vi "LINC Create Command Definition.vi"(8 "error in (no error)":errorcluster, 10 "path":path, 11 "LINC session":refnum<class "LINC.lvclass">) -> (0 "error out":errorcluster, 3 "dup LINC session":refnum<class "LINC.lvclass">)   [LabVIEW 2018, in "STEPkgDriver_LINC.lvlib" / "LINC.lvclass"]
uses:
  LINC.lvclass
  STEPkgDriver_LINC.lvlib
  LINC Global Mode.ctl
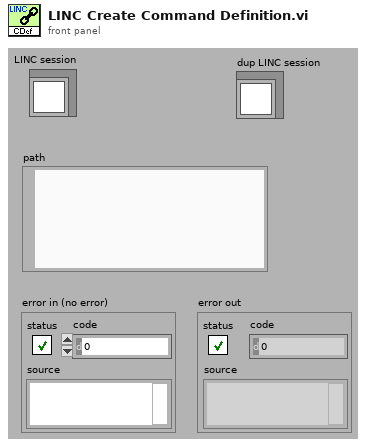
[diagram p1: front panel]
types:
  T1 = typedef "STEPkgDriver_LINC.lvlib/LINC Global Mode.ctl" = enum16{"INIT", "CLEAR", "ADD_PKT_HDR", "ADD_PKT", "GET_PKT_NAMES", "GET_PKT_DESC", "GET_PKT_HDR", "GET_PKT", "SET_PKT", "SET_DATA", "SIM_EN", "SIM_DS"}
  T2 = typedef "STEPkgDriver_LINC.lvlib/LINC Format Prototype.ctl" = cluster{"type":string, "bit offset":i32, "bit size":i32, "format":string, "unit":string, "description":string, "state values":i64[], "states":string[], "max":string, "min":string, "default":string, "array":bool, "bit element size":i32, "poly bound":dbl[], "poly scale":cluster{"coefficients":dbl[]}[], "labview size":i32, "simulate":bool, "ID":bool, "required":bool}
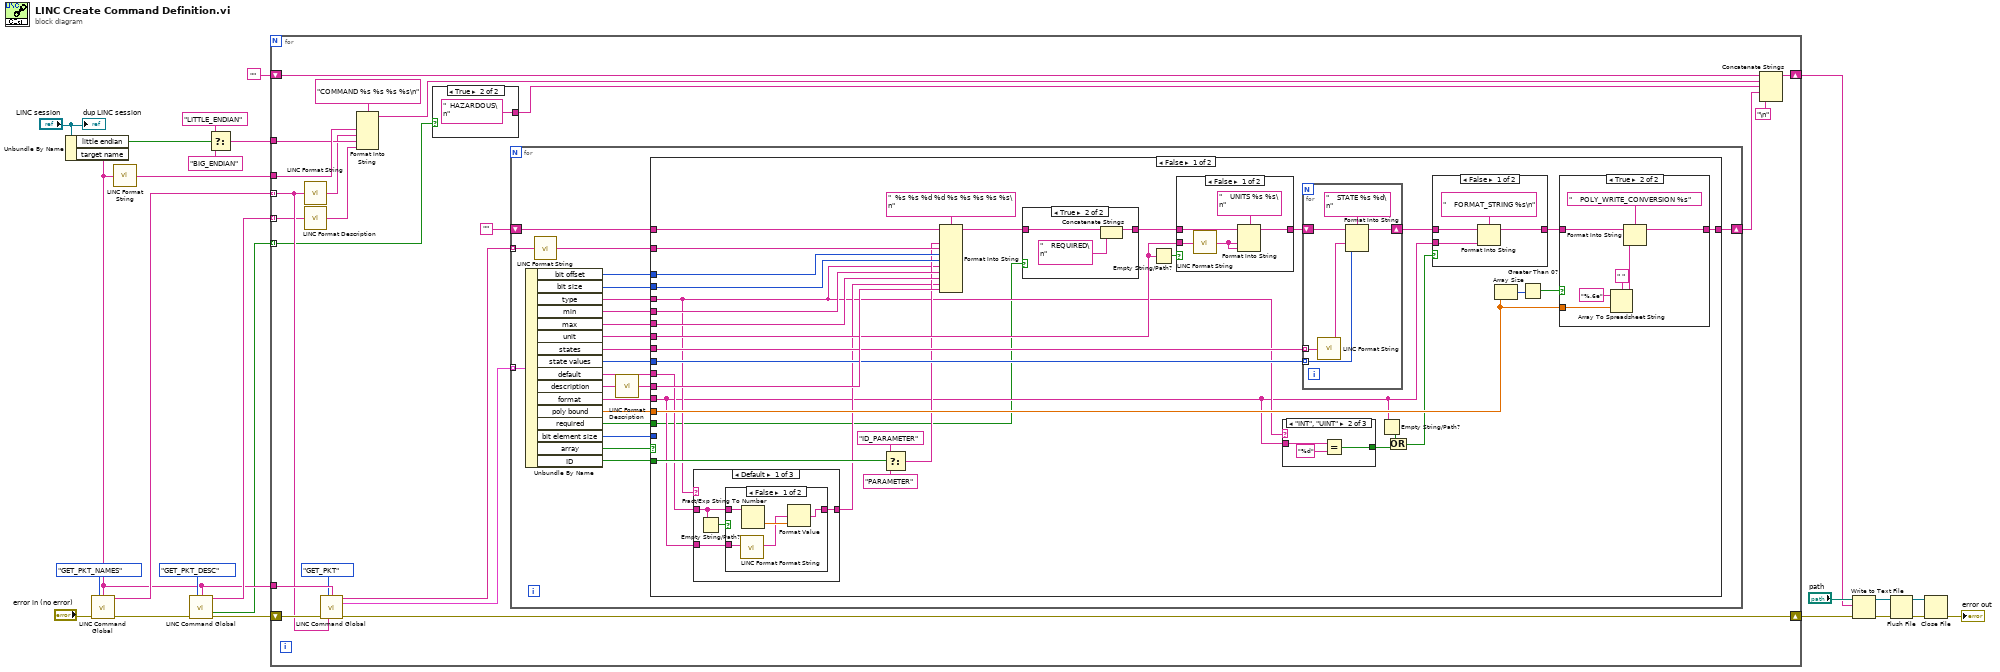
[diagram p0: block diagram]
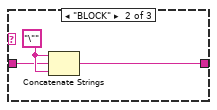
[diagram p5: hidden frame]
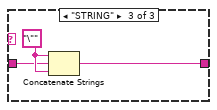
[diagram p6: hidden frame]
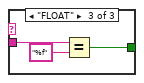
[diagram p8: hidden frame]
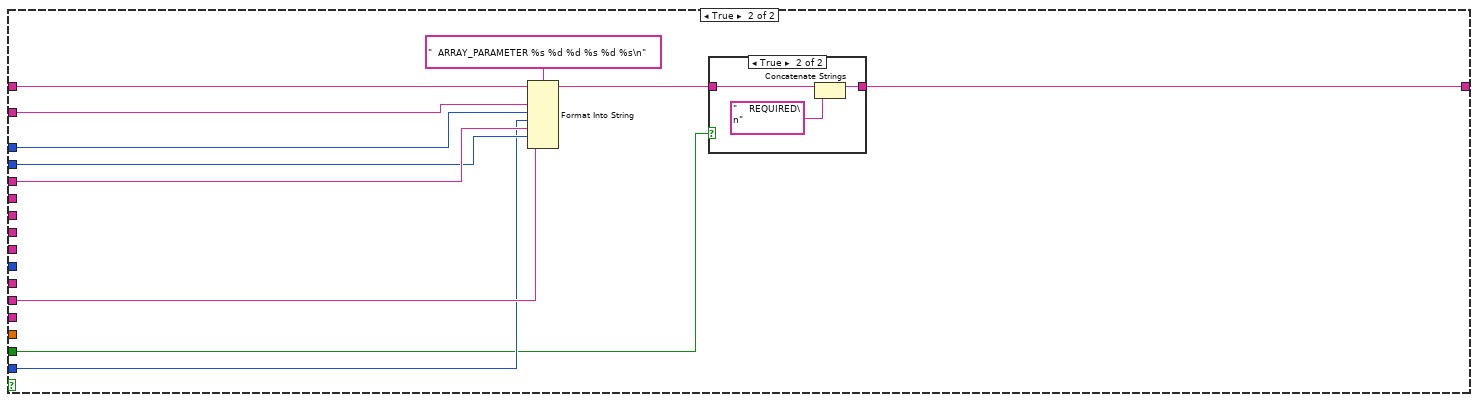
[diagram p12: hidden frame]
diagram:
  n1 = Unbundle By Name("LINC session") -> ("little endian"=w4:bool, "target name"=w2:string)
  n2 = call "LINC Command Global.vi"("mode"=LINC_Global_Mode."GET_PKT_NAMES", "target name"=w2, "error in (no error)"="error in (no error)") -> ("values out"=w17:string[], "error out"=w14:errorcluster)  [unwired: 8 in, 3 out]
  n3 = call "LINC Format String.vi"("string in"=w2) -> ("string out"=w3:string)
  n4 = call "LINC Command Global.vi"("mode"=LINC_Global_Mode."GET_PKT_DESC", "target name"=w2, "error in (no error)"=w14) -> ("values out"=w13:string[], "hazardous out"=w1:bool[], "error out"=w9:errorcluster)  [unwired: 8 in, 2 out]
  n5 = Select(t="LITTLE_ENDIAN", s=w4, f="BIG_ENDIAN") -> (s? t:f=w5:string)
  n6 = for {
    tunnel: w3 -> [w45]
    tunnel: w13 -> [w26] mode=indexing
    shift-right: [w36] -> w8
    shift-left: "" -> [w41]
    shift-right: [w39] -> w16
    shift-left: w9 -> [w40]
    tunnel: w17 -> [w30] mode=indexing
    tunnel: w2 -> [w38]
    tunnel: w5 -> [w32]
    tunnel: w1 -> [w29] mode=indexing
    n7 = call "LINC Format String.vi"("string in"=w30) -> ("string out"=w31:string)
    n8 = call "LINC Format Description.vi"("string in"=w26) -> ("string out"=w25:string)
    n9 = call "LINC Command Global.vi"("mode"=LINC_Global_Mode."GET_PKT", "target name"=w38, "error in (no error)"=w40, "packet name"=w30) -> ("values out"=w34:string[], "item formats out"=w35:T2[], "error out"=w39:errorcluster)  [unwired: 7 in, 2 out]
    n10 = Format Into String(format string="COMMAND %s %s %s %s\n", w45, w31, w32, w25) -> (resulting string=w28:string)  [unwired: 2 in, 1 out]
    n11 = case shown="True" w29 {
      tunnel: [_ "  HAZARDOUS\n" ("format string")] -> w27
      frame False {
      }
      frame True {
      }
    }
    n12 = for {
      shift-right: [w67] -> w37
      shift-left: "" -> [w68]
      tunnel: w34 -> [w50] mode=indexing
      tunnel: w35 -> [w63] mode=indexing
      n13 = Unbundle By Name(w63) -> ("bit offset"=w60:i32, "bit size"=w59:i32, "type"=w64:string, "min"=w56:string, "max"=w55:string, "unit"=w66:string, "states"=w65:string[], "state values"=w62:i64[], "default"=w48:string, "description"=w52:string, "format"=w53:string, "poly bound"=w57:dbl[], "required"=w47:bool, "bit element size"=w58:i32, "array"=w61:bool, "ID"=w54:bool)
      n14 = call "LINC Format String.vi"("string in"=w50) -> ("string out"=w49:string)
      n15 = call "LINC Format Description.vi"("string in"=w52) -> ("string out"=w51:string)
      n16 = case shown="False" w61 {
        tunnel: w68 -> [w100 w162]
        tunnel: [w72 w154] -> w67
        tunnel: w53 -> [w73 _]
        tunnel: w51 -> [w98 w161]
        tunnel: w56 -> [w95 _]
        tunnel: w55 -> [w94 _]
        tunnel: w66 -> [w93 _]
        tunnel: w65 -> [w92 _]
        tunnel: w49 -> [w84 w160]
        tunnel: w64 -> [w75 w159]
        tunnel: w60 -> [w91 w158]
        tunnel: w62 -> [w90 _]
        tunnel: w59 -> [w89 w157]
        tunnel: w58 -> [_ w156]
        tunnel: w57 -> [w85 _]
        tunnel: w54 -> [w83 _]
        tunnel: w48 -> [w74 _]
        tunnel: w47 -> [w69 w153]
        frame False {
          n17 = case shown="Default" w75 {
            tunnel: w74 -> [w108 w117 w120]
            tunnel: [w107 w116 w119] -> w78
            tunnel: w73 -> [w106 _ _]
            frame Default {
              n18 = Empty String/Path?(string/path=w108) -> (empty?=w109:bool)
              n19 = case shown="False" w109 {
                tunnel: w106 -> [w114 _]
                tunnel: w108 -> [w113 w115]
                tunnel: [w110 w115] -> w107
                frame False {
                  n20 = call "LINC Format Format String.vi"("format in"=w114) -> ("format out"=w111:string)  [unwired: 10 in]
                  n21 = Fract/Exp String To Number(string=w113) -> (number=w112:dbl)  [unwired: 3 in, 1 out]
                  n22 = Format Value(format string=w111, value (0)=w112) -> (output string=w110:string)  [unwired: 1 in]
                }
                frame True {
                }
              }
            }
            frame "BLOCK" {
              w118 = "\"" ("string")
              n23 = Concatenate Strings(w118, w117, w118) -> (w116:string)
            }
            frame "STRING" {
              w121 = "\"" ("string")
              n24 = Concatenate Strings(w121, w120, w121) -> (w119:string)
            }
          }
          n25 = Select(t="ID_PARAMETER", s=w83, f="PARAMETER") -> (s? t:f=w81:string)
          n26 = Format Into String(format string="  %s %s %d %d %s %s %s %s %s\n", initial string=w100, w81, w84, w91, w89, w75, w95, w94, w78, w98) -> (resulting string=w71:string)  [unwired: 1 in, 1 out]
          n27 = case shown="True" w69 {
            tunnel: w71 -> [w102 w104]
            tunnel: [w102 w103] -> w70
            frame False {
            }
            frame True {
              n28 = Concatenate Strings(w104, "    REQUIRED\n" ("format string")) -> (w103:string)
            }
          }
          n29 = Empty String/Path?(string/path=w93) -> (empty?=w97:bool)
          n30 = case shown="False" w97 {
            tunnel: w70 -> [w139 w141]
            tunnel: [w138 w141] -> w96
            tunnel: w93 -> [w137 _]
            frame False {
              n31 = call "LINC Format String.vi"("string in"=w137) -> ("string out"=w136:string)
              n32 = Format Into String(format string="    UNITS %s %s\n", initial string=w139, w136, w136) -> (resulting string=w138:string)  [unwired: 1 in, 1 out]
            }
            frame True {
            }
          }
          n33 = case shown="\"INT\", \"UINT\"" w75 {
            tunnel: w73 -> [_ w123 w126]
            tunnel: [_ w122 w125] -> w76
            frame Default {
            }
            frame "INT", "UINT" {
              n34 = Equal?(x=w123, y="%d") -> (x = y?=w122:bool)
            }
            frame "FLOAT" {
              n35 = Equal?(x=w126, y="%f") -> (x = y?=w125:bool)
            }
          }
          n36 = for {
            shift-right: [w151] -> w99
            shift-left: w96 -> [w152]
            tunnel: w92 -> [w148] mode=indexing
            tunnel: w90 -> [w149] mode=indexing
            n37 = call "LINC Format String.vi"("string in"=w148) -> ("string out"=w147:string)
            n38 = Format Into String(format string="    STATE %s %d\n", initial string=w152, w147, w149) -> (resulting string=w151:string)  [unwired: 1 in, 1 out]
          }
          n39 = Empty String/Path?(string/path=w73) -> (empty?=w77:bool)
          n40 = Or(x=w77, y=w76) -> (x .or. y?=w80:bool)
          n41 = case shown="False" w80 {
            tunnel: w99 -> [w144 w146]
            tunnel: [w143 w146] -> w86
            tunnel: w73 -> [w142 _]
            frame False {
              n42 = Format Into String(format string="    FORMAT_STRING %s\n", initial string=w144, w142) -> (resulting string=w143:string)  [unwired: 1 in, 1 out]
            }
            frame True {
            }
          }
          n43 = Array Size(array=w85) -> (size(s)=w87:i32)
          n44 = Greater Than 0?(x=w87) -> (x > 0?=w88:bool)
          n45 = case shown="True" w88 {
            tunnel: w86 -> [w128 w134]
            tunnel: [w128 w133] -> w72
            tunnel: w85 -> [_ w130]
            frame False {
            }
            frame True {
              n46 = Array To Spreadsheet String(delimiter (Tab)=" ", array=w130, 3:"%.6e" ("format string")) -> (spreadsheet string=w129:string)
              n47 = Format Into String(format string="    POLY_WRITE_CONVERSION %s", initial string=w134, w129) -> (resulting string=w133:string)  [unwired: 1 in, 1 out]
            }
          }
        }
        frame True {
          n48 = Format Into String(format string="  ARRAY_PARAMETER %s %d %d %s %d %s\n", initial string=w162, w160, w158, w156, w159, w157, w161) -> (resulting string=w155:string)  [unwired: 1 in, 1 out]
          n49 = case shown="True" w153 {
            tunnel: w155 -> [w164 w166]
            tunnel: [w164 w165] -> w154
            frame False {
            }
            frame True {
              n50 = Concatenate Strings(w166, "    REQUIRED\n" ("format string")) -> (w165:string)
            }
          }
        }
      }
    }
    n51 = Concatenate Strings(w41, w28, w27, w37, "\n") -> (w36:string)
  }
  n52 = Write to Text File(file (use dialog)="path", text=w8, error in=w16) -> (refnum out=w22:refnum<file>, error out=w23:errorcluster)  [unwired: 2 out]
  n53 = Flush File(refnum=w22, error in=w23) -> (refnum out=w20:refnum<file>, error out=w21:errorcluster)
  n54 = Close File(refnum=w20, error in=w21) -> (error out=→"error out":errorcluster)  [unwired: 1 out]
  "dup LINC session" <- "LINC session"
